vi "UDP_receive_001.vi"() -> ()   [LabVIEW 2019]
panel:
  out "data out":string
  in  "stop":bool
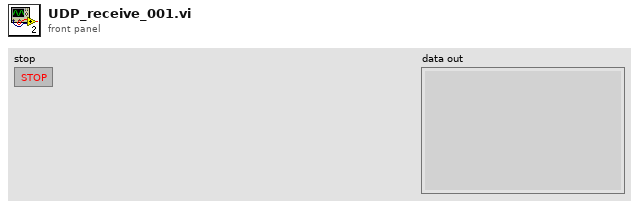
[diagram p1: front panel]
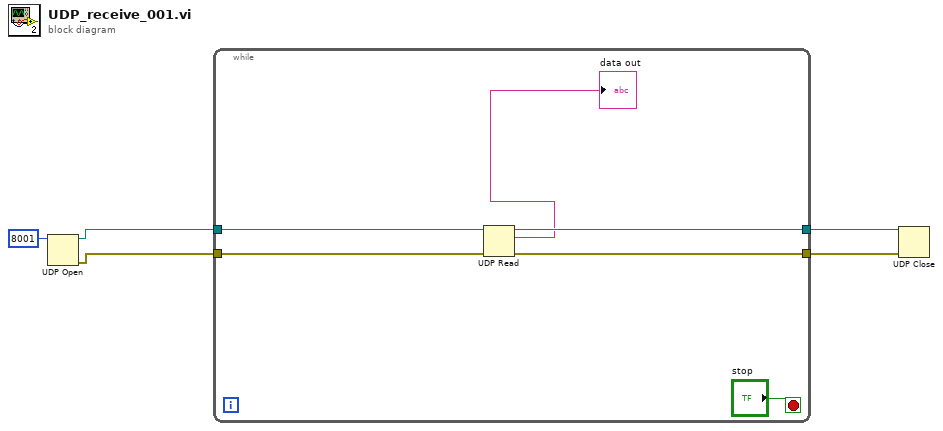
[diagram p0: block diagram]
diagram:
  n1 = UDP Open(11:u16 8001 ("port")) -> (port=w5:refnum<k16>, 0:w3:errorcluster)  [unwired: 4 in, 1 out]
  n2 = while {
    tunnel: w5 -> [w10]
    tunnel: [w9] -> w4
    tunnel: w3 -> [w8]
    tunnel: [w7] -> w2
    stop <- "stop" stop-if-true
    n3 = UDP Read(connection ID=w10, 8:w8) -> (data out=→"data out":string, error out=w7:errorcluster, 3:w9:refnum<k16>)  [unwired: 2 in, 2 out]
  }
  n4 = UDP Close(connection ID=w4, 8:w2) -> ()  [unwired: 2 out]
